vi "test_SessionInitializationErrors_InitializeSessions_NothingAddedToConnectionMap.vi"(8 "error in":errorcluster) -> (0 "error out":errorcluster, 2 "result":string, 3 "pass":bool)   [LabVIEW 2020, in "MeasurementServerTests.lvlib"]
uses:
  MeasurementServerTests.lvlib
  Runtime/Clients/Session Management V1/Session Reservation/Connection with Session.ctl
  Runtime/Clients/Session Management V1/Session Reservation/Connection.ctl
  Runtime/Clients/Session Management V1/Session Reservation/Pin Type.ctl
  Runtime/Clients/Session Management V1/Session Reservation/Initialize and Close Session Behavior.ctl
  f6a09b6e-aad0-4c3a-b0f0-322e876417ba.vi
  a956f7ee-c7e9-4639-884c-f4265dae6ecf.vi
  bf15b356-c08f-4dd9-8162-1f405dfb48eb.vi
  bf15b356-c08f-4dd9-8162-1f405dfb48eb.vi/7fd45821-cfd3-468e-85e7-fb0eb05eda95.vi
  Helpers/Fake Session Factory/Fake Session Factory.lvclass
  C:/dev/measurementlink-labview/Source/Runtime/Sessions/Instrument Sessions/ISession Factory/ISession Factory.lvclass
  Runtime/Clients/Session Management V1/Session Reservation/Initialize Sessions with Retry.vi
  Runtime/Clients/Session Management V1/Session Reservation/Get Connections Impl.vi
  Runtime/Clients/Session Management V1/Session Reservation/Session Reservation.lvclass
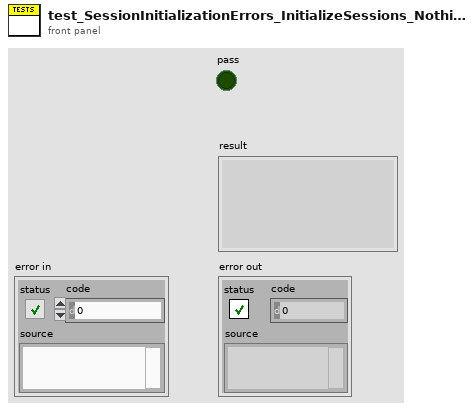
[diagram p1: front panel]
types:
  T1 = typedef "NI Session Management V1 Client.lvlib/Session Reservation.lvclass/Initialize and Close Session Behavior.ctl" = enum16{"Auto", "Initialize and Close", "Attach and Detach", "Initialize and Detach", "Attach and Close"}
  T2 = typedef "NI Session Management V1 Client.lvlib/Session Reservation.lvclass/Pin Type.ctl" = enum16{"DUT and System Pins", "System Pins"}
  T3 = typedef "NI Session Management V1 Client.lvlib/Session Reservation.lvclass/Connection with Session.ctl" = cluster{"connection":T4, "session":variant}
  T4 = typedef "NI Session Management V1 Client.lvlib/Session Reservation.lvclass/Connection.ctl" = cluster{"pin or relay name":string, "site":i32, "instrument type id":string, "channel":string}
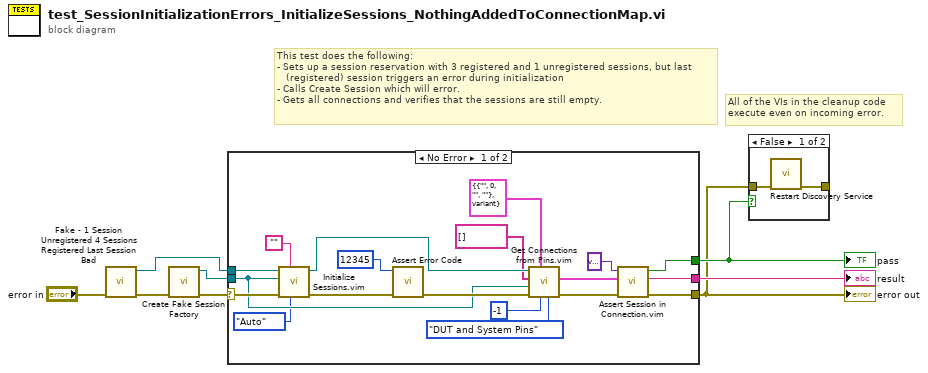
[diagram p0: block diagram]
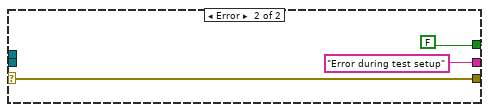
[diagram p2: hidden frame]
diagram:
  # "All of the VIs in the cleanup code\nexecute even on incoming error."
  # "This test does the following:\n- Sets up a session reservation with 3 registered and 1 unregistered sessions, but last\n   (registered) session triggers an error during initialization\n- Calls Create Session which will error. \n- Gets all connections and verifies that the sessions are still empty."
  n1 = call "Fake - 1 Session Unregistered 4 Sessions Registered Last Session Bad.vi"("error in"="error in") -> ("error out"=w2:errorcluster, "session reservation out"=w1:refnum<class "Session Reservation.lvclass">)  [unwired: 9 in]
  n2 = call "Create Fake Session Factory.vi"("error in"=w2) -> ("error out"=w5:errorcluster, "fake session factory out"=w4:refnum<class "Fake Session Factory.lvclass">)  [unwired: 9 in]
  n3 = case shown="No Error" w5 {
    selector: w5 -> [w25 w27]
    tunnel: [w19 w27] -> w6
    tunnel: [w12 FALSE] -> w7
    tunnel: [w17 "Error during test setup" ("f")] -> w8
    tunnel: w4 -> [w10 _]
    tunnel: w1 -> [w26 _]
    frame No Error {
      n4 = call "Initialize Sessions.vim"("initialize and close session behavior"=Initialize_and_Close_Session_Behavior."Auto", "session type"="", "error in"=w25, "session factory"=w10, "session reservation in"=w26) -> ("error out"=w16:errorcluster, "session reservation out"=w23:refnum<class "Session Reservation.lvclass">)  [unwired: 3 in, 2 out]
      n5 = call "Assert Error Code.vi"("error in"=w16, "expected error code"=12345) -> ("error out"=w15:errorcluster)  [unwired: 7 in, 2 out]
      n6 = call "Get Connections from Pins.vim"("pin type"=Pin_Type."DUT and System Pins", "site"=-1, "connection type"=T3 {"connection"={"pin or relay name"="", "site"=0, "instrument type id"="", "channel"=""}, "session"=variant}, "error in"=w15, "session factory"=w10, "pin or relay names"=string[] [], "session reservation in"=w23) -> ("error out"=w19:errorcluster, "connections"=w18:T3[])  [unwired: 2 in, 1 out]
      n7 = call "Assert Session in Connection.vim"("actual connections"=w18, "expected session"=variant) -> ("result"=w17:string, "pass"=w12:bool)  [unwired: 8 in]
    }
    frame Error {
    }
  }
  "error out" <- w6
  "pass" <- w7
  "result" <- w8
  n8 = case shown="False" w7 {
    tunnel: w6 -> [w31 _]
    tunnel: [w30 _] -> _
    frame False {
      n9 = call "Restart Discovery Service.vi"("error in"=w31) -> ("error out"=w30:errorcluster)  [unwired: 10 in]
    }
    frame True {
    }
  }
